vi "Panel Get Loads.vi"(2 "file path (dialog if empty)":path) -> (6 "Load Type Out":string(combo), 8 "Nominal Load  Weight Out":string(combo))   [LabVIEW 2009]
uses:
  <vilib>/Utility/file.llb/Read From Spreadsheet File (string).vi
panel:
  in  "Nominal Load  Weight (Select or Enter Value)":string(combo)
  in  "Load Type (Select or Enter Value)":string(combo)
  in  "stop":bool
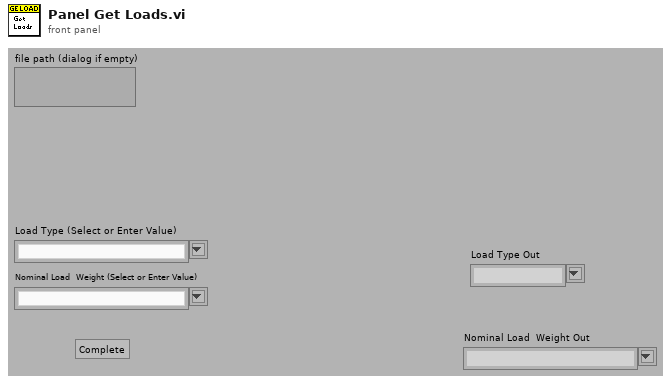
[diagram p1: front panel]
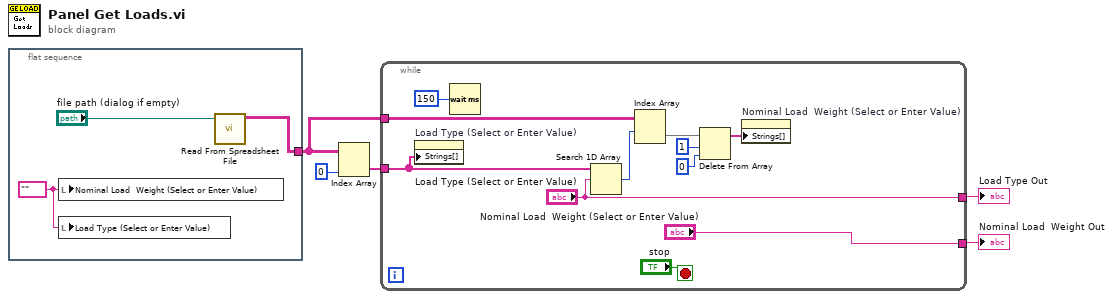
[diagram p0: block diagram]
diagram:
  n1 = flat-sequence {
    tunnel: [w6] -> w1
    frame #0 {
      w8 = "" ("Load Type (Select or Enter Value)")
      n2 = local write "Nominal Load  Weight (Select or Enter Value)"(w8) -> ()
      n3 = local write "Load Type (Select or Enter Value)"(w8) -> ()
      n4 = call-poly <vilib>:"Read From Spreadsheet File.vi"("file path (dialog if empty)"="file path (dialog if empty)") -> ("all rows"=w6:string[][])  [unwired: 6 in, 4 out]
    }
  }
  n5 = Index Array(array=w1, index (col)=0 ("disabled index (col)")) -> (element=w4:string[])  [unwired: 1 in]
  n6 = while {
    tunnel: w4 -> [w17]
    tunnel: ["Load Type (Select or Enter Value)"] -> w3
    tunnel: w1 -> [w15]
    tunnel: ["Nominal Load  Weight (Select or Enter Value)"] -> w2
    stop <- "stop" stop-if-true
    n7 = property on="Load Type (Select or Enter Value)" class="CmbBox"("Strings[]"=w17) -> ()  [unwired: 2 in, 2 out]
    n8 = Wait (ms)(milliseconds to wait=u32 150) -> ()  [unwired: 1 out]
    n9 = Search 1D Array(1D array=w17, element="Load Type (Select or Enter Value)") -> (index of element=w14:i32)  [unwired: 1 in]
    n10 = Index Array(array=w15, index (row)=w14) -> (element=w13:string[])  [unwired: 1 in]
    n11 = Delete From Array(array=w13, length=1, index=0) -> (array with subset deleted=w10:string[])  [unwired: 1 out]
    n12 = property on="Nominal Load  Weight (Select or Enter Value)" class="CmbBox"("Strings[]"=w10) -> ()  [unwired: 2 in, 2 out]
  }
  "Load Type Out" <- w3
  "Nominal Load  Weight Out" <- w2
